vi "Set Trigger.vi"(8 "error in (no error)":errorcluster, 10 "Source":string, 11 "Camera in":refnum<class "Camera.lvclass">) -> (0 "error out":errorcluster, 3 "Camera":refnum<class "Camera.lvclass">)   [LabVIEW 2020, in "Camera.lvclass"]
uses:
  Camera.lvclass
  Camera.lvclass/Camera.ctl
  Check Not Disconnected.vi
  <vilib>/Utility/error.llb/Error Cluster From Error Code.vi
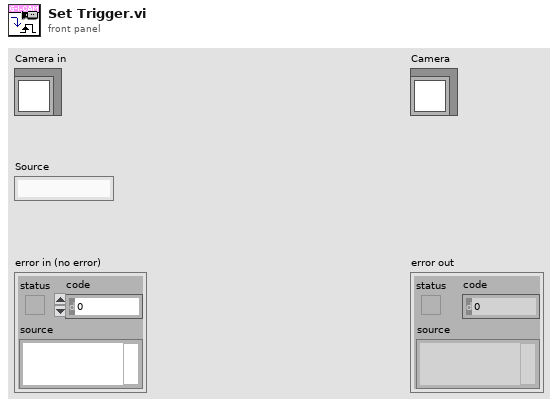
[diagram p1: front panel]
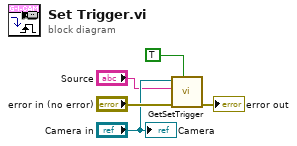
[diagram p0: block diagram]
diagram:
  n1 = call "GetSetTrigger.vi"("Set"=TRUE, "error in (no error)"="error in (no error)", "Source"="Source", "Camera in"="Camera in") -> ("error out"=→"error out":errorcluster)  [unwired: 6 in, 1 out]
  "Camera" <- "Camera in"
